vi "GradientBoostingRegressor.vi"(8 "error in":errorcluster) -> (0 "error out":errorcluster, 3 "out":refnum<class "GradientBoostingRegressor.lvclass">)   [LabVIEW 2020]
doc: "Gradient Boosting for regression.\n\n GB builds an additive model in a forward stage-wise fashion;\n it allows for the optimization of arbitrary differentiable loss functions.\n In each stage a regression tree is fit on the negative gradient of the\n given loss function.\n\n Read more in the :ref:`User Guide <gradient_boosting>`.\n\n Parameters\n ----------\n loss : {'ls', 'lad', 'huber', 'quantile'}, default='ls'\n Loss function to be optimized. 'ls' refers to least squares\n regression. 'lad' (least absolute deviation) is a highly robust\n loss function solely based on order information of the input\n variables. 'huber' is a combination of the two. 'quantile'\n allows quantile regression (use `alpha` to specify the quantile).\n\n learning_rate : float, default=0.1\n Learning rate shrinks the contribution of each tree by `learning_rate`.\n There is a trade-off between learning_rate and n_estimators.\n\n n_estimators : int, default=100\n The number of boosting stages to perform. Gradient boosting\n is fairly robust to over-fitting so a large number usually\n results in better performance.\n\n subsample : float, default=1.0\n The fraction of samples to be used for fitting the individual base\n learners. If smaller than 1.0 this results in Stochastic Gradient\n Boosting. `subsample` interacts with the parameter `n_estimators`.\n Choosing `subsample < 1.0` leads to a reduction of variance\n and an increase in bias.\n\n criterion : {'friedman_mse', 'mse', 'mae'}, default='friedman_mse'\n The function to measure the quality of a split. Supported criteria\n are \"friedman_mse\" for the mean squared error with improvement\n score by Friedman, \"mse\" for mean squared error, and \"mae\" for\n the mean absolute error. The default value of \"friedman_mse\" is\n generally the best as it can provide a better approximation in\n some cases.\n\n .. versionadded:: 0.18\n .. deprecated:: 0.24\n `criterion='mae'` is deprecated and will be removed in version\n 1.1 (renaming of 0.26). The correct way of minimizing the absolute\n error is to use `loss='lad'` instead.\n\n min_samples_split : int or float, default=2\n The minimum number of samples required to split an internal node:\n\n - If int, then consider `min_samples_split` as the minimum number.\n - If float, then `min_samples_split` is a fraction and\n `ceil(min_samples_split * n_samples)` are the minimum\n number of samples for each split.\n\n .. versionchanged:: 0.18\n Added float values for fractions.\n\n min_samples_leaf : int or float, default=1\n The minimum number of samples required to be at a leaf node.\n A split point at any depth will only be considered if it leaves at\n least ``min_samples_leaf`` training samples in each of the left and\n right branches. This may have the effect of smoothing the model,\n especially in regression.\n\n - If int, then consider `min_samples_leaf` as the minimum number.\n - If float, then `min_samples_leaf` is a fraction and\n `ceil(min_samples_leaf * n_samples)` are the minimum\n number of samples for each node.\n\n .. versionchanged:: 0.18\n Added float values for fractions.\n\n min_weight_fraction_leaf : float, default=0.0\n The minimum weighted fraction of the sum total of weights (of all\n the input samples) required to be at a leaf node. Samples have\n equal weight when sample_weight is not provided.\n\n max_depth : int, default=3\n Maximum depth of the individual regression estimators. The maximum\n depth limits the number of nodes in the tree. Tune this parameter\n for best performance; the best value depends on the interaction\n of the input variables.\n\n min_impurity_decrease : float, default=0.0\n A node will be split if this split induces a decrease of the impurity\n greater than or equal to this value.\n\n The weighted impurity decrease equation is the following::\n\n N_t / N * (impurity - N_t_R / N_t * right_impurity\n - N_t_L / N_t * left_impurity)\n\n where ``N`` is the total number of samples, ``N_t`` is the number of\n samples at the current node, ``N_t_L`` is the number of samples in the\n left child, and ``N_t_R`` is the number of samples in the right child.\n\n ``N``, ``N_t``, ``N_t_R`` and ``N_t_L`` all refer to the weighted sum,\n if ``sample_weight`` is passed.\n\n .. versionadded:: 0.19\n\n min_impurity_split : float, default=None\n Threshold for early stopping in tree growth. A node will split\n if its impurity is above the threshold, otherwise it is a leaf.\n\n .. deprecated:: 0.19\n ``min_impurity_split`` has been deprecated in favor of\n ``min_impurity_decrease`` in 0.19. The default value of\n ``min_impurity_split`` has changed from 1e-7 to 0 in 0.23 and it\n will be removed in 1.0 (renaming of 0.25).\n Use ``min_impurity_decrease`` instead.\n\n init : estimator or 'zero', default=None\n An estimator object that is used to compute the initial predictions.\n ``init`` has to provide :term:`fit` and :term:`predict`. If 'zero', the\n initial raw predictions are set to zero. By default a\n ``DummyEstimator`` is used, predicting either the average target value\n (for loss='ls'), or a quantile for the other losses.\n\n random_state : int, RandomState instance or None, default=None\n Controls the random seed given to each Tree estimator at each\n boosting iteration.\n In addition, it controls the random permutation of the features at\n each split (see Notes for more details).\n It also controls the random spliting of the training data to obtain a\n validation set if `n_iter_no_change` is not None.\n Pass an int for reproducible output across multiple function calls.\n See :term:`Glossary <random_state>`.\n\n max_features : {'auto', 'sqrt', 'log2'}, int or float, default=None\n The number of features to consider when looking for the best split:\n\n - If int, then consider `max_features` features at each split.\n - If float, then `max_features` is a fraction and\n `int(max_features * n_features)` features are considered at each\n split.\n - If \"auto\", then `max_features=n_features`.\n - If \"sqrt\", then `max_features=sqrt(n_features)`.\n - If \"log2\", then `max_features=log2(n_features)`.\n - If None, then `max_features=n_features`.\n\n Choosing `max_features < n_features` leads to a reduction of variance\n and an increase in bias.\n\n Note: the search for a split does not stop until at least one\n valid partition of the node samples is found, even if it requires to\n effectively inspect more than ``max_features`` features.\n\n alpha : float, default=0.9\n The alpha-quantile of the huber loss function and the quantile\n loss function. Only if ``loss='huber'`` or ``loss='quantile'``.\n\n verbose : int, default=0\n Enable verbose output. If 1 then it prints progress and performance\n once in a while (the more trees the lower the frequency). If greater\n than 1 then it prints progress and performance for every tree.\n\n max_leaf_nodes : int, default=None\n Grow trees with ``max_leaf_nodes`` in best-first fashion.\n Best nodes are defined as relative reduction in impurity.\n If None then unlimited number of leaf nodes.\n\n warm_start : bool, default=False\n When set to ``True``, reuse the solution of the previous call to fit\n and add more estimators to the ensemble, otherwise, just erase the\n previous solution. See :term:`the Glossary <warm_start>`.\n\n validation_fraction : float, default=0.1\n The proportion of training data to set aside as validation set for\n early stopping. Must be between 0 and 1.\n Only used if ``n_iter_no_change`` is set to an integer.\n\n .. versionadded:: 0.20\n\n n_iter_no_change : int, default=None\n ``n_iter_no_change`` is used to decide if early stopping will be used\n to terminate training when validation score is not improving. By\n default it is set to None to disable early stopping. If set to a\n number, it will set aside ``validation_fraction`` size of the training\n data as validation and terminate training when validation score is not\n improving in all of the previous ``n_iter_no_change`` numbers of\n iterations.\n\n .. versionadded:: 0.20\n\n tol : float, default=1e-4\n Tolerance for the early stopping. When the loss is not improving\n by at least tol for ``n_iter_no_change`` iterations (if set to a\n number), the training stops.\n\n .. versionadded:: 0.20\n\n ccp_alpha : non-negative float, default=0.0\n Complexity parameter used for Minimal Cost-Complexity Pruning. The\n subtree with the largest cost complexity that is smaller than\n ``ccp_alpha`` will be chosen. By default, no pruning is performed. See\n :ref:`minimal_cost_complexity_pruning` for details.\n\n .. versionadded:: 0.22\n\n Attributes\n ----------\n feature_importances_ : ndarray of shape (n_features,)\n The impurity-based feature importances.\n The higher, the more important the feature.\n The importance of a feature is computed as the (normalized)\n total reduction of the criterion brought by that feature. It is also\n known as the Gini importance.\n\n Warning: impurity-based feature importances can be misleading for\n high cardinality features (many unique values). See\n :func:`sklearn.inspection.permutation_importance` as an alternative.\n\n oob_improvement_ : ndarray of shape (n_estimators,)\n The improvement in loss (= deviance) on the out-of-bag samples\n relative to the previous iteration.\n ``oob_improvement_[0]`` is the improvement in\n loss of the first stage over the ``init`` estimator.\n Only available if ``subsample < 1.0``\n\n train_score_ : ndarray of shape (n_estimators,)\n The i-th score ``train_score_[i]`` is the deviance (= loss) of the\n model at iteration ``i`` on the in-bag sample.\n If ``subsample == 1`` this is the deviance on the training data.\n\n loss_ : LossFunction\n The concrete ``LossFunction`` object.\n\n init_ : estimator\n The estimator that provides the initial predictions.\n Set via the ``init`` argument or ``loss.init_estimator``.\n\n estimators_ : ndarray of DecisionTreeRegressor of shape (n_estimators, 1)\n The collection of fitted sub-estimators.\n\n n_classes_ : int\n The number of classes, set to 1 for regressors.\n\n .. deprecated:: 0.24\n Attribute ``n_classes_`` was deprecated in version 0.24 and\n will be removed in 1.1 (renaming of 0.26).\n\n n_estimators_ : int\n The number of estimators as selected by early stopping (if\n ``n_iter_no_change`` is specified). Otherwise it is set to\n ``n_estimators``.\n\n n_features_ : int\n The number of data features.\n\n max_features_ : int\n The inferred value of max_features.\n\n See Also\n --------\n HistGradientBoostingRegressor : Histogram-based Gradient Boosting\n Classification Tree.\n sklearn.tree.DecisionTreeRegressor : A decision tree regressor.\n sklearn.tree.RandomForestRegressor : A random forest regressor.\n\n Notes\n -----\n The features are always randomly permuted at each split. Therefore,\n the best found split may vary, even with the same training data and\n ``max_features=n_features``, if the improvement of the criterion is\n identical for several splits enumerated during the search of the best\n split. To obtain a deterministic behaviour during fitting,\n ``random_state`` has to be fixed.\n\n \nAvailable methods:\nFit\nPredict\nScore\nGet Attributes\nGet Params\nSet Params"
uses:
  GradientBoostingRegressor.lvclass
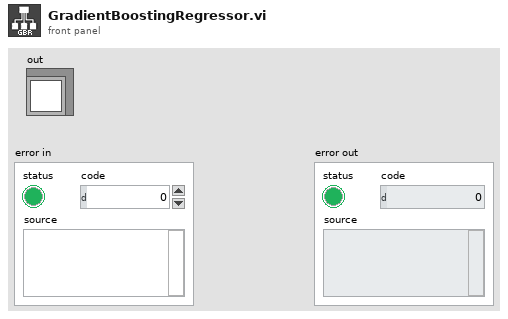
[diagram p1: front panel]
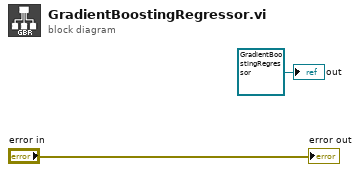
[diagram p0: block diagram]
diagram:
  "out" <- refnum<class "GradientBoostingRegressor.lvclass"> refnum ("model")
  "error out" <- "error in"
